vi "采配水参数设置.vi"() -> ()   [LabVIEW 2016, in "采配水.lvlib"]
uses:
  <vilib>/Utility/config.llb/NI_LVConfig.lvlib
panel:
  in  "自动补水":bool
  out "配水时间":dbl=1800.0
  in  "布尔":bool
  out "沉淀时间":dbl=1800.0
  out "进样超时时间":dbl=300.0
  out "润洗时间":dbl=60.0
  out "排空时间":dbl=60.0
  # "参数设置"
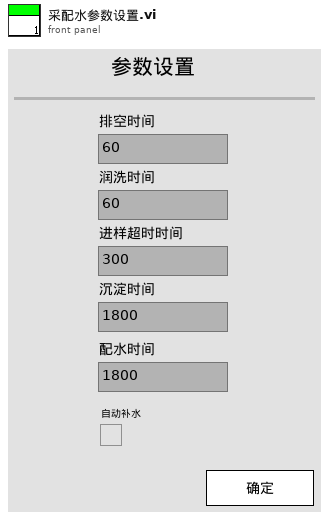
[diagram p1: front panel]
types:
  T1 = cluster{"排空时间":dbl, "润洗时间":dbl, "进样超时时间":dbl, "沉淀时间":dbl, "配水时间":dbl}
  T2 = typedef "NI_LVConfig.lvlib/Config Data RefNum.ctl" = refnum<k1>
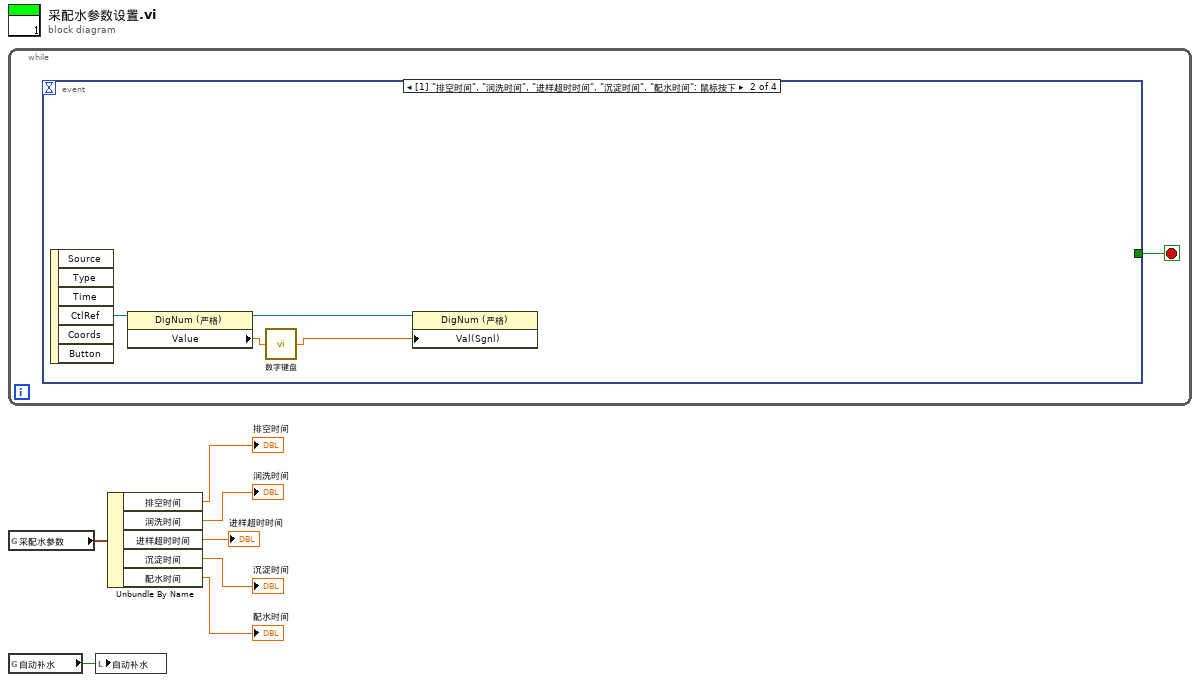
[diagram p0: block diagram]
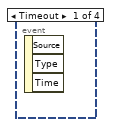
[diagram p2: hidden frame]
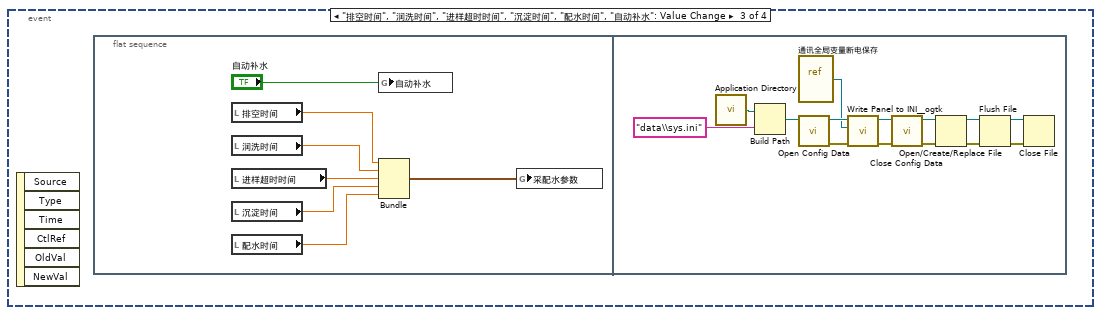
[diagram p3: hidden frame]
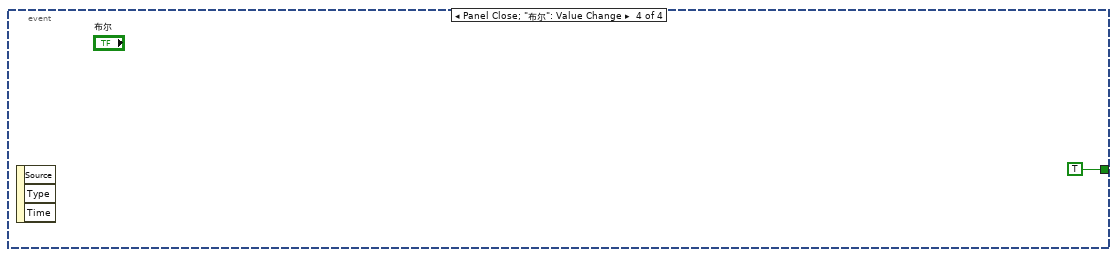
[diagram p4: hidden frame]
diagram:
  n1 = while {
    stop <- w8 stop-if-true
    n2 = event shown="[1] \"排空时间\", \"润洗时间\", \"进样超时时间\", \"沉淀时间\", \"配水时间\": 鼠标按下" {
      selector: _ -> [_ _ _ _]
      dyn-events: _ -> [_ _ _ _]
      timeout: _ -> [_ _ _ _]
      tunnel: [_ _ _ TRUE] -> w8
      event Timeout {
        n3 = event-data() -> ()  [unwired: 1 in, 3 out]
      }
      event "排空时间", "润洗时间", "进样超时时间", "沉淀时间", "配水时间": Mouse Down {
        n4 = event-data() -> ("CtlRef"=w12:refnum<vi>)  [unwired: 1 in, 5 out]
        n5 = property class="DigNum (严格)"(reference=w12) -> (reference out=w9:refnum<vi>, "Value"=w11:dbl)  [unwired: 1 in, 1 out]
        n6 = call "数字键盘.vi"("OldNumber"=w11) -> ("NewNumber"=w10:dbl)
        n7 = property class="DigNum (严格)"(reference=w9, "Val(Sgnl)"=w10) -> ()  [unwired: 1 in, 2 out]
      }
      event "排空时间", "润洗时间", "进样超时时间", "沉淀时间", "配水时间", "自动补水": Value Change {
        n8 = event-data() -> ()  [unwired: 1 in, 6 out]
        n9 = flat-sequence {
          frame #0 {
            n10 = local read "排空时间"() -> (w19:dbl)
            n11 = local read "润洗时间"() -> (w18:dbl)
            n12 = local read "进样超时时间"() -> (w17:dbl)
            n13 = local read "沉淀时间"() -> (w16:dbl)
            n14 = local read "配水时间"() -> (w14:dbl)
            n15 = global write "通讯全局变量断电保存.vi" "自动补水"("自动补水") -> ()
            n16 = Bundle("排空时间"=w19, "润洗时间"=w18, "进样超时时间"=w17, "沉淀时间"=w16, "配水时间"=w14) -> (w15:T1)  [unwired: 1 in]
            n17 = global write "通讯全局变量断电保存.vi" "采配水参数"(w15) -> ()
          }
          frame #1 {
            n18 = call <vilib>:"Application Directory.vi"() -> ("Application Directory"=w33:path)
            n19 = Build Path(base path=w33, name or relative path="data\\sys.ini" ("名称或相对路径")) -> (appended path=w31:path)
            n20 = vi-ref "通讯全局变量断电保存.vi"() -> (w29:refnum<vi>)
            n21 = call <vilib>:"Open Config Data.vi"("configuration file path"=w31) -> ("error out"=w27:errorcluster, "refnum"=w30:T2)  [unwired: 8 in, 1 out]
            n22 = call <userlib>:"Write Panel to INI__ogtk.vi"("error in (no error)"=w27, "VI ref"=w29, "refnum"=w30) -> ("error out"=w26:errorcluster, "refnum out"=w28:T2)  [unwired: 7 in]
            n23 = call <vilib>:"Close Config Data.vi"("error in (no error)"=w26, "refnum"=w28) -> ("error out"=w21:errorcluster, "file path"=w20:path)  [unwired: 8 in]
            n24 = Open/Create/Replace File(file path (use dialog)=w20, error in=w21) -> (refnum out=w24:refnum<file>, error out=w25:errorcluster)  [unwired: 4 in, 1 out]
            n25 = Flush File(refnum=w24, error in=w25) -> (refnum out=w23:refnum<file>, error out=w22:errorcluster)
            n26 = Close File(refnum=w23, error in=w22) -> ()  [unwired: 2 out]
          }
        }
      }
      event Panel Close; "布尔": Value Change {
        n27 = event-data() -> ()  [unwired: 1 in, 3 out]
      }
    }
  }
  n28 = global read "通讯全局变量断电保存.vi" "采配水参数"() -> (w7:T1)
  n29 = global read "通讯全局变量断电保存.vi" "自动补水"() -> (w1:bool)
  n30 = local write "自动补水"(w1) -> ()
  n31 = Unbundle By Name(w7) -> ("排空时间"=→"排空时间":dbl, "润洗时间"=→"润洗时间":dbl, "进样超时时间"=→"进样超时时间":dbl, "沉淀时间"=→"沉淀时间":dbl, "配水时间"=→"配水时间":dbl)
